vi "Start Inline Rx.vi"(8 "error in (no error)":errorcluster, 9 "framework iteration":u64=1, 10 "Dispatcher Interface in":refnum<class "Dispatcher Interface.lvclass">, 11 "Scheduler in":refnum<class "Scheduler.lvclass">) -> (0 "error out":errorcluster, 2 "Dispatcher Interface out":refnum<class "Dispatcher Interface.lvclass">, 3 "Scheduler out":refnum<class "Scheduler.lvclass">)   [LabVIEW 2017, in "DSF Core.lvlib" / "Scheduler.lvclass"]
uses:
  Scheduler.lvclass
  Timing/Plugin Timing Group.lvclass
  Interfaces/Dispatcher/Dispatcher Interface.lvclass
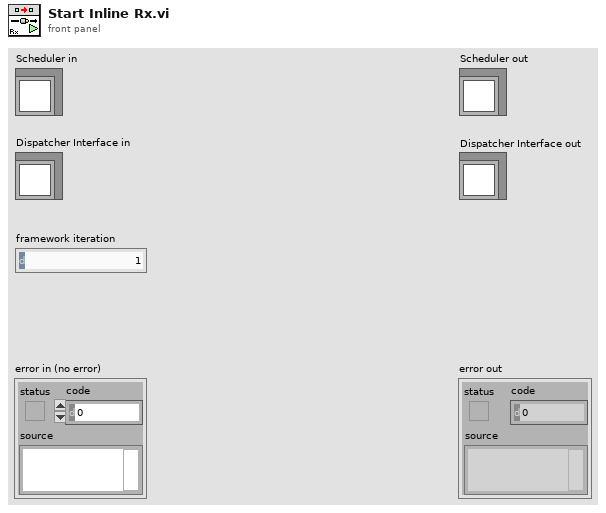
[diagram p1: front panel]
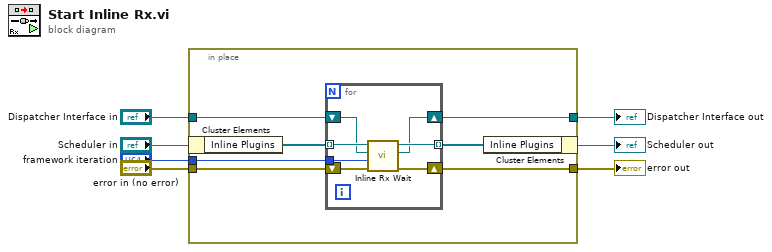
[diagram p0: block diagram]
diagram:
  n1 = in-place {
    in-place-border: "framework iteration" -> [w13]
    in-place-border: "Dispatcher Interface in" -> [w12]
    in-place-border: [w11] -> w3
    in-place-border: "error in (no error)" -> [w10]
    in-place-border: [w9] -> w1
    n2 = in-place-cluster #1("Scheduler in") -> ("Inline Plugins"=w14:refnum<class "Plugin Timing Group.lvclass">[])
    n3 = for {
      tunnel: w14 -> [w18] mode=indexing
      tunnel: w13 -> [w20]
      shift-right: [w15] -> w11
      shift-left: w12 -> [w16]
      shift-right: [w21] -> w9
      shift-left: w10 -> [w19]
      tunnel: [w17] -> w8 mode=indexing
      n4 = call "Inline Rx Wait.vi"("error in (no error)"=w19, 9:w20, "Dispatcher Interface in"=w16, "Plugin Timing Group in"=w18) -> ("error out"=w21:errorcluster, "Dispatcher Interface out"=w15:refnum<class "Dispatcher Interface.lvclass">, "Plugin Timing Group out"=w17:refnum<class "Plugin Timing Group.lvclass">)  [unwired: 5 in]
    }
    n5 = in-place-cluster #1("Inline Plugins"=w8) -> (→"Scheduler out":refnum<class "Scheduler.lvclass">)
  }
  "error out" <- w1
  "Dispatcher Interface out" <- w3
